vi "Untitled 1.vi"   [LabVIEW 2012]
uses:
  <vilib>/NXT/Hardware/Plugins/Tetrix DC Motor/TetrixDCMotorAddress.ctl
  <vilib>/NXT/Block Support/NXT_OutputPort.ctl
  <vilib>/NXT/NXTIO Xnodes/NXTIONodeSubVIs/TETRIX IO Move DC Motors.vi
  <vilib>/NXT/NXTIO Xnodes/NXTIONodeSubVIs/TETRIX IO Check Battery.vi
  <vilib>/NXT/NXTIO Xnodes/NXTIONodeSubVIs/NXTStopMotors.vi
  <vilib>/NXT/NXTIO Xnodes/NXTIONodeSubVIs/TETRIX IO Stop DC Motors.vi
  <vilib>/NXT/Subs/LVHSConnector.ctl
  <vilib>/NXT/NXTIO Xnodes/AddressXNode/NXTIOAddress.xnode
  LabVIEW Data/NXTRobotics/Projects/testdrive/testdrive.lvrbt
  <vilib>/NXT/NXTIO Xnodes/NXTIOXNode/NXTIO.xnode
  <vilib>/NXT/LegoClasses/BrickReference/BrickReference.lvclass
types:
  T1 = typedef "TetrixDCMotorAddress.ctl" = i16
  T2 = cluster{"TetrixDCMotor":T1, "TetrixDCMotor 2":T1}
  T3 = typedef "LVHSConnector.ctl" = refnum<class "BrickReference.lvclass">
  T4 = typedef "FTC ControllerState.ctl" = cluster{"Left X":i8, "Left Y":i8, "Right X":i8, "Right Y":i8, "Button Encoding 9-12":u8, "Button Encoding 1-8":u8, "POV":T5}
  T5 = typedef "FTC POVState.ctl" = i8
  T6 = typedef "NXT_OutputPort.ctl" = u8
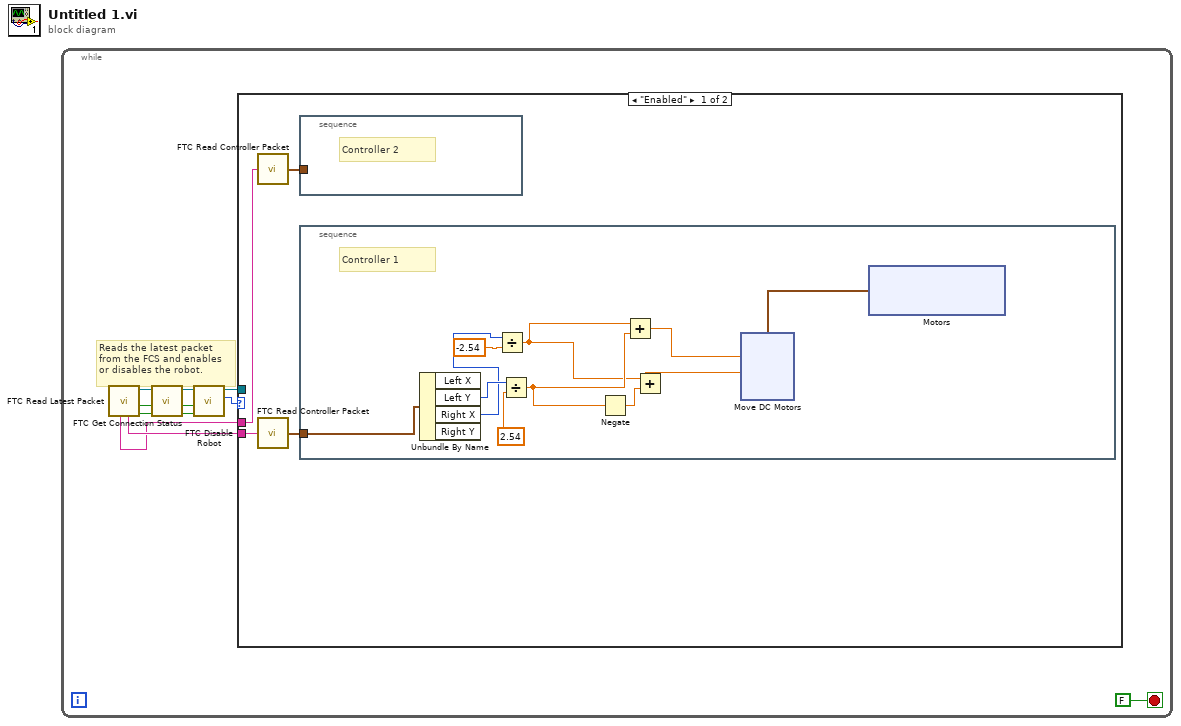
[diagram p0: block diagram]
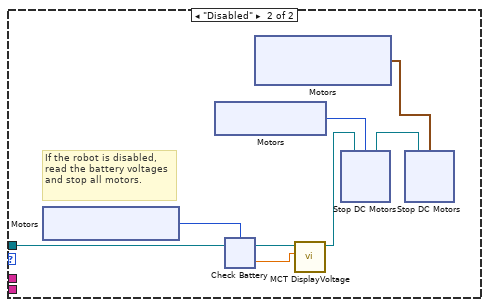
[diagram p2: hidden frame]
diagram:
  n1 = while {
    stop <- FALSE stop-if-true
    # "Reads the latest packet\nfrom the FCS and enables\nor disables the robot."
    n2 = call <vilib>:"FTC Read Latest Packet.vi"() -> ("Packet Received?"=w9:bool, "Stopped?"=w6:bool, "NXT"=w8:T3, "Controller 1"=w11:string, "Controller 2"=w10:string)  [unwired: 6 in, 1 out]
    n3 = call <vilib>:"FTC Get Connection Status.vi"("Packet Received?"=w9, "Stopped?"=w6, "NXT"=w8) -> ("Online?"=w3:bool, "Stopped?"=w4:bool, "NXT"=w5:T3)  [unwired: 5 in]
    n4 = call <vilib>:"FTC Disable Robot.vi"("Online?"=w3, "Stopped?"=w4, "NXT"=w5) -> ("Enabled?"=w7:enum16{"Disabled", "Enabled"}, "NXT"=w2:T3)  [unwired: 3 in]
    n5 = case "disableCase" shown="\"Enabled\"" w7 {
      tunnel: w11 -> [w15 _]
      tunnel: w10 -> [w14 _]
      tunnel: w2 -> [_ w45]
      frame "Enabled" {
        n6 = call <vilib>:"FTC Read Controller Packet.vi"("Packet"=w14) -> ("Controller State"=w12:T4)  [unwired: 4 in]
        n7 = call <vilib>:"FTC Read Controller Packet.vi"("Packet"=w15) -> ("Controller State"=w13:T4)  [unwired: 4 in]
        n8 = stacked-sequence "controller2Actions" {
          tunnel: w12 -> [_]
          frame #0 {
            # "Controller 2"
          }
        }
        n9 = stacked-sequence "controller1Actions" {
          tunnel: w13 -> [w25]
          frame #0 {
            # "Controller 1"
            n10 = Unbundle By Name(w25) -> ("Left Y"=w18:i8, "Right X"=w17:i8)  [unwired: 2 out]
            n11 = Divide(x=w17, y=-2.54) -> (x/y=w16:dbl)
            n12 = Divide(x=w18, y=2.54) -> (x/y=w19:dbl)
            n13 = Negate(x=w19) -> (-x=w20:dbl)
            n14 = Add(x=w16, y=w19) -> (x+y=w22:dbl)
            n15 = Add(x=w16, y=w20) -> (x+y=w21:dbl)
            n16 = xnode ("Motors")() -> ("Motor"=w26:cluster{"TetrixDCMotor":T1, "TetrixDCMotor":T1})
            n17 = xnode ("Move DC Motors")("Power/Speed 2"=w21, "Power/Speed 1"=w22, "Motors"=w26) -> ()  [unwired: 1 in, 1 out]
          }
        }
      }
      frame "Disabled" {
        # "If the robot is disabled, read the battery voltages and stop all motors."
        n18 = xnode ("Motors")() -> ("Motor"=w44:T1)
        n19 = xnode "Motors"() -> ("Motor"=w41:T6)
        n20 = xnode ("Check Battery")("Motors"=w44, "NXT"=w45) -> ("Voltage 1"=w43:sgl, "NXT"=w42:T3)
        n21 = xnode "Motors"() -> ("Motor"=w39:cluster{"TetrixDCMotor":T1, "TetrixDCMotor":T1})
        n22 = call <vilib>:"MCT DisplayVoltage.vi"("Motor Voltage"=w43, "NXT"=w42) -> ("NXT"=w40:T3)  [unwired: 9 in]
        n23 = xnode "Stop DC Motors"("Motors"=w41, "NXT"=w40) -> ("NXT"=w38:T3)
        n24 = xnode "Stop DC Motors"("Motors"=w39, "NXT"=w38) -> ()  [unwired: 1 out]
      }
    }
  }
